vi "Close_StreamRefs.vi"(7 "CloseDestinationStream [T]":bool=TRUE, 8 "error in (no error)":errorcluster, 11 "HttpContent in":refnum<class "HttpContent.lvclass">) -> (0 "error out":errorcluster, 3 "HttpContent out":refnum<class "HttpContent.lvclass">)   [LabVIEW 2018, in "HttpClient_NET.lvlib" / "HttpContent.lvclass"]
uses:
  HttpContent.lvclass
  HttpContent.lvclass/HttpContent.ctl
  Accessors/Read NET_DestinationStream.vi
  Accessors/Read NET_SourceStream.vi
  Accessors/Read NET_StreamTask.vi
  Accessors/Read NET_StreamCancellationSource.vi
  Accessors/Write NET_DestinationStream.vi
  Accessors/Write NET_SourceStream.vi
  Accessors/Write NET_StreamTask.vi
  Accessors/Write NET_StreamCancellationSource.vi
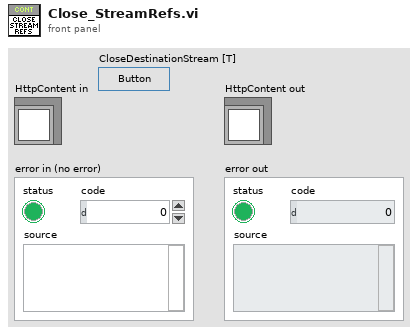
[diagram p1: front panel]
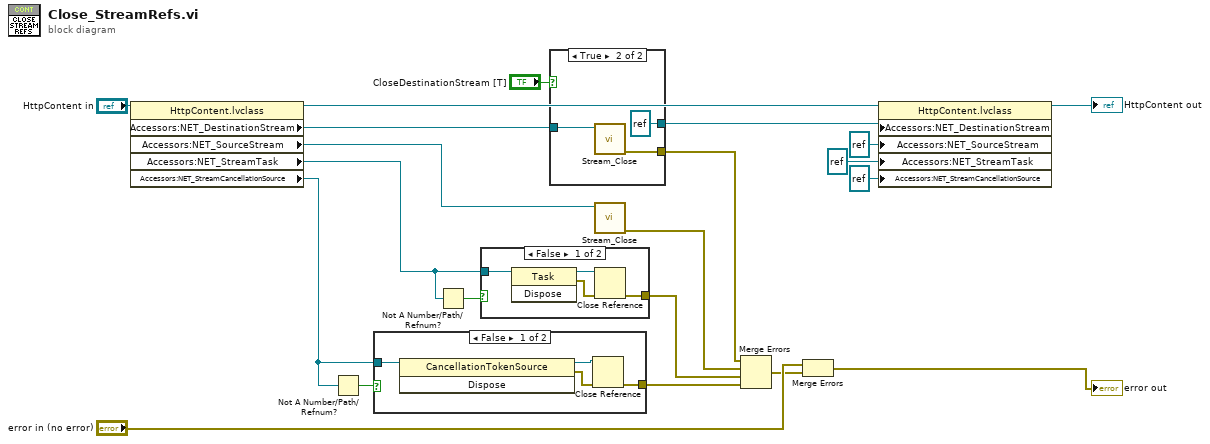
[diagram p0: block diagram]
diagram:
  n1 = property class="HttpContent.lvclass"(reference="HttpContent in") -> (reference out=w12:refnum<class "HttpContent.lvclass">, "Accessors:NET_DestinationStream"=w13:refnum<k24>, "Accessors:NET_SourceStream"=w14:refnum<k24>, "Accessors:NET_StreamTask"=w10:refnum<k24>, "Accessors:NET_StreamCancellationSource"=w7:refnum<k24>)  [unwired: 1 in, 1 out]
  n2 = Not A Number/Path/Refnum?(number/path/refnum=w7) -> (NaN/Path/Refnum?=w8:bool)
  n3 = case shown="False" w8 {
    tunnel: [w25 _] -> w15
    tunnel: w7 -> [w22 _]
    frame False {
      n4 = invoke class="CancellationTokenSource" method="Dispose"(reference=w22) -> (reference out=w24:refnum<k24>, error out=w23:errorcluster)  [unwired: 2 in, 1 out]
      n5 = Close Reference(reference=w24, error in (no error)=w23) -> (error out=w25:errorcluster)
    }
    frame True {
    }
  }
  n6 = Not A Number/Path/Refnum?(number/path/refnum=w10) -> (NaN/Path/Refnum?=w9:bool)
  n7 = case shown="False" w9 {
    tunnel: [w29 _] -> w16
    tunnel: w10 -> [w26 _]
    frame False {
      n8 = invoke class="Task" method="Dispose"(reference=w26) -> (reference out=w27:refnum<k24>, error out=w28:errorcluster)  [unwired: 2 in, 1 out]
      n9 = Close Reference(reference=w27, error in (no error)=w28) -> (error out=w29:errorcluster)
    }
    frame True {
    }
  }
  n10 = case shown="True" "CloseDestinationStream [T]" {
    tunnel: [_ w33] -> w18
    tunnel: w13 -> [w30 w32]
    tunnel: [w30 refnum<k24> refnum ("NET_DestinationStream")] -> w1
    frame False {
    }
    frame True {
      n11 = call "Stream_Close.vi"("Stream"=w32) -> ("error out"=w33:errorcluster)  [unwired: 10 in]
    }
  }
  n12 = call "Stream_Close.vi"("Stream"=w14) -> ("error out"=w17:errorcluster)  [unwired: 10 in]
  n13 = Merge Errors(w18, w17, w16, w15) -> (w19:errorcluster)
  n14 = Merge Errors("error in (no error)", w19) -> (→"error out":errorcluster)
  n15 = property class="HttpContent.lvclass"(reference=w12, "Accessors:NET_DestinationStream"=w1, "Accessors:NET_SourceStream"=refnum<k24> refnum ("NET_SourceStream"), "Accessors:NET_StreamTask"=refnum<k24> refnum ("NET_StreamTask"), "Accessors:NET_StreamCancellationSource"=refnum<k24> refnum ("NET_StreamCancellationSource")) -> (reference out=→"HttpContent out":refnum<class "HttpContent.lvclass">)  [unwired: 1 in, 1 out]
